vi "RP - READ MAC CONF FILE.vi"(8 "error in (no error)":errorcluster, 11 "Path":path) -> (0 "error out":errorcluster, 2 "RP2 MAC":string, 3 "RP1 MAC":string)   [LabVIEW 2021]
uses:
  <vilib>/Utility/config.llb/Write Key (String).vi
  <vilib>/Utility/config.llb/Read Key (String).vi
  <vilib>/Utility/config.llb/NI_LVConfig.lvlib
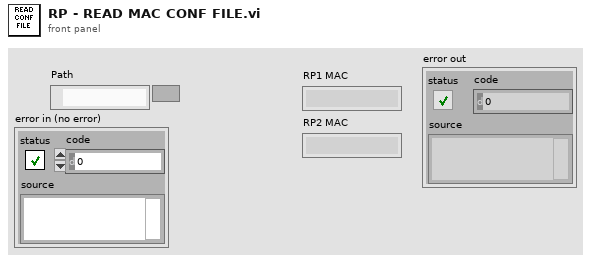
[diagram p1: front panel]
types:
  T1 = typedef "NI_LVConfig.lvlib/Config Data RefNum.ctl" = refnum<k1>
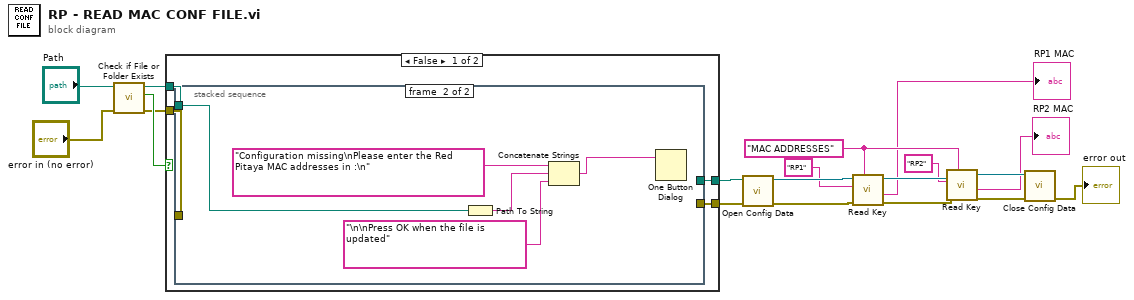
[diagram p0: block diagram]
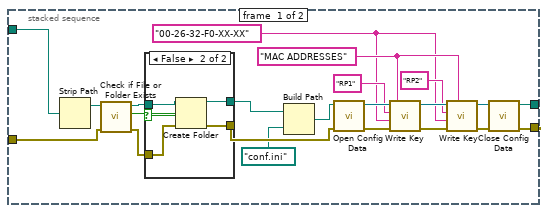
[diagram p2: hidden frame]
diagram:
  w8 = "MAC ADDRESSES" ("section")
  n1 = call <vilib>:"Check if File or Folder Exists.vi"("error in (no error)"="error in (no error)", "path"="Path") -> ("error out"=w15:errorcluster, "file or folder exists?"=w17:bool, "dup path"=w18:path)  [unwired: 7 in]
  n2 = case shown="False" w17 {
    tunnel: w18 -> [w23 w57]
    tunnel: w15 -> [w22 w58]
    tunnel: [w21 w58] -> w4
    tunnel: [w20 w57] -> w5
    frame False {
      n3 = stacked-sequence {
        tunnel: w23 -> [w45 w56]
        tunnel: [w31 _] -> w20
        tunnel: w22 -> [w30 _]
        tunnel: [w27 _] -> w21
        frame #0 {
          w35 = "MAC ADDRESSES" ("section")
          w32 = "00-26-32-F0-XX-XX"
          n4 = Strip Path(path=w45) -> (stripped path=w44:path)  [unwired: 1 out]
          n5 = call <vilib>:"Check if File or Folder Exists.vi"("error in (no error)"=w30, "path"=w44) -> ("error out"=w29:errorcluster, "file or folder exists?"=w43:bool, "dup path"=w42:path)  [unwired: 7 in]
          n6 = case shown="False" w43 {
            tunnel: w42 -> [w47 w48]
            tunnel: [w47 w51] -> w26
            tunnel: w29 -> [w46 w50]
            tunnel: [w46 w49] -> w28
            frame True {
            }
            frame False {
              n7 = Create Folder(path (use dialog)=w48, error in=w50) -> (created path=w51:path, error out=w49:errorcluster)  [unwired: 1 in, 1 out]
            }
          }
          n8 = Build Path(base path=w26, name or relative path=path "conf.ini") -> (appended path=w25:path)
          n9 = call <vilib>:"Open Config Data.vi"("error in (no error)"=w28, "configuration file path"=w25) -> ("error out"=w41:errorcluster, "refnum"=w40:T1)  [unwired: 7 in, 1 out]
          n10 = call-poly <vilib>:"Write Key.vi"("section"=w35, "error in (no error)"=w41, "value"=w32, "key"="RP1", "refnum"=w40) -> ("error out"=w38:errorcluster, "refnum out"=w39:T1)  [unwired: 4 in, 1 out]
          n11 = call-poly <vilib>:"Write Key.vi"("section"=w35, "error in (no error)"=w38, "value"=w32, "key"="RP2", "refnum"=w39) -> ("error out"=w36:errorcluster, "refnum out"=w37:T1)  [unwired: 4 in, 1 out]
          n12 = call <vilib>:"Close Config Data.vi"("error in (no error)"=w36, "refnum"=w37) -> ("error out"=w27:errorcluster, "file path"=w31:path)  [unwired: 8 in]
        }
        frame #1 {
          n13 = Path To String(path=w56) -> (string=w55:string)
          n14 = Concatenate Strings("Configuration missing\nPlease enter the Red Pitaya MAC addresses in :\n" ("message"), w55, "\n\nPress OK when the file is updated" ("string")) -> (w54:string)
          n15 = One Button Dialog(message=w54) -> ()  [unwired: 1 in, 1 out]
        }
      }
    }
    frame True {
    }
  }
  n16 = call <vilib>:"Open Config Data.vi"("error in (no error)"=w4, "configuration file path"=w5) -> ("error out"=w10:errorcluster, "refnum"=w9:T1)  [unwired: 7 in, 1 out]
  n17 = call-poly <vilib>:"Read Key.vi"("section"=w8, "error in (no error)"=w10, "key"="RP1", "refnum"=w9) -> ("error out"=w12:errorcluster, "value"=→"RP1 MAC":string, "refnum out"=w11:T1)  [unwired: 4 in, 1 out]
  n18 = call-poly <vilib>:"Read Key.vi"("section"=w8, "error in (no error)"=w12, "key"="RP2", "refnum"=w11) -> ("error out"=w14:errorcluster, "value"=→"RP2 MAC":string, "refnum out"=w13:T1)  [unwired: 4 in, 1 out]
  n19 = call <vilib>:"Close Config Data.vi"("error in (no error)"=w14, "refnum"=w13) -> ("error out"=→"error out":errorcluster)  [unwired: 8 in, 1 out]
